vi "subCallConfigTx.vi"(0 "session handle":refnum<k15>, 5 "Tx Parameters":T1={"Tx IQ Sampling\nRate [s/sec]"=200000.0, "Tx Frequency [Hz]"=433920000.0, "Tx Gain [dB]"=0.0, "Tx Antenna"=""} {"Tx Gain [dB]" format="%#.6p"; "Tx Frequency [Hz]" format="%#.6p"; "Tx IQ Sampling\nRate [s/sec]" format="%#.6p"}, 11 "error in":errorcluster) -> (4 "session handle out":refnum<k15>, 6 "Actual Tx Parameters":T1 {"Tx Gain [dB]" format="%#.6p"; "Tx Frequency [Hz]" format="%#.6p"; "Tx IQ Sampling\nRate [s/sec]" format="%#.6p"}, 15 "error out":errorcluster)   [LabVIEW 2013]
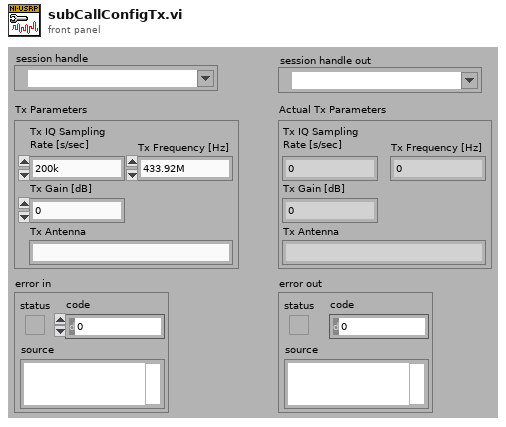
[diagram p1: front panel]
types:
  T1 = cluster{"Tx IQ Sampling\nRate [s/sec]":dbl, "Tx Frequency [Hz]":dbl, "Tx Gain [dB]":dbl, "Tx Antenna":string}
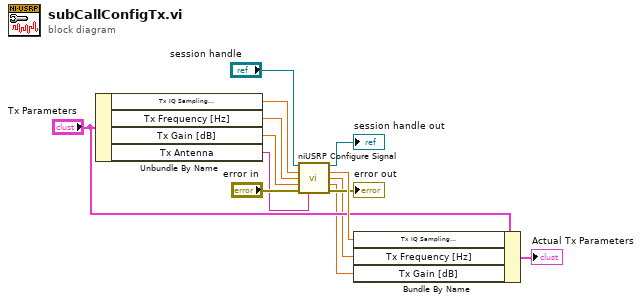
[diagram p0: block diagram]
diagram:
  n1 = Unbundle By Name("Tx Parameters") -> ("Tx IQ Sampling\nRate [s/sec]"=w11:dbl, "Tx Frequency [Hz]"=w5:dbl, "Tx Gain [dB]"=w4:dbl, "Tx Antenna"=w1:string)
  n2 = call <instrlib>:"niUSRP Configure Signal.vi"("session handle"="session handle", "IQ rate"=w11, "carrier frequency"=w5, "gain"=w4, "error in (no error)"="error in", "active antenna"=w1) -> ("session handle out"=→"session handle out":refnum<k15>, "coerced IQ rate"=w13:dbl, "coerced carrier frequency"=w3:dbl, "coerced gain"=w2:dbl, "error out"=→"error out":errorcluster)  [unwired: 5 in]
  n3 = Bundle By Name(cluster="Tx Parameters", "Tx IQ Sampling\nRate [s/sec]"=w13, "Tx Frequency [Hz]"=w3, "Tx Gain [dB]"=w2) -> (→"Actual Tx Parameters":T1)
